vi "Launch Action - TDMS Writer Segmented.vi"(8 "error in (no error)":errorcluster, 9 "CAN Configurations":T2[](array[typedef]) {"Sample Rate (Hz)" format="%#_13g"}, 10 "DAQ AI Configurations":T1[](array[typedef]) {"Terminal Config" items=["Default"=-1, "RSE"=10083, "NRSE"=10078, "Differential"=10106, "Pseudodifferential"=12529]; "Min (V)" format="%#_13g"; "Max (V)" format="%#_13g"; "Sample Rate (Hz)" format="%#_13g"}, 11 "Log file path":path) -> (0 "error out":errorcluster)   [LabVIEW 2021, in "XNET-CAN-Signal-Logger.lvlib"]
uses:
  XNET-CAN-Signal-Logger.lvlib
  Typedef/Def-CAN Port Configuration.ctl
  Typedef/Def-DAQ AI Configuration.ctl
  Action - TDMS Writer.vi
  Global Variables.vi
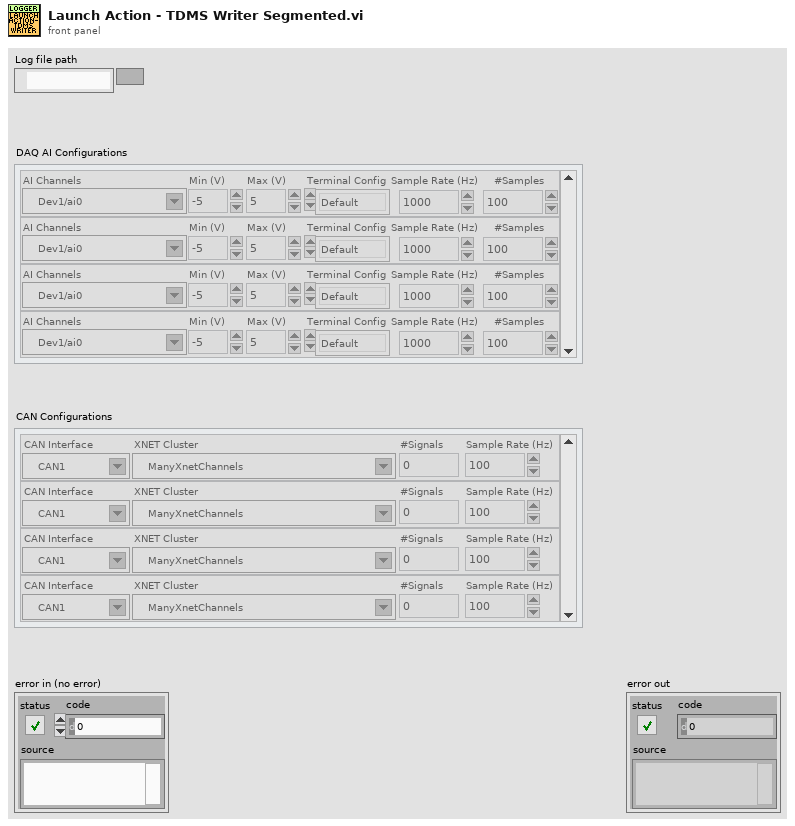
[diagram p1: front panel]
types:
  T1 = typedef "XNET-CAN-Signal-Logger.lvlib/Def-DAQ AI Configuration.ctl" = cluster{"AI Channels":tag, "Min (V)":dbl, "Max (V)":dbl, "Terminal Config":i32, "Sample Rate (Hz)":dbl, "#Samples":i32}
  T2 = typedef "XNET-CAN-Signal-Logger.lvlib/Def-CAN Port Configuration.ctl" = cluster{"CAN Interface":refnum<k21>, "XNET Cluster":refnum<k21>, "#Signals":i32, "Sample Rate (Hz)":dbl}
  T3 = enum16{"open", "open or create", "create or replace", "create", "open (read-only)"}
  T4 = typedef "XNET-CAN-Signal-Logger.lvlib/Def-FGV Data Type.ctl" = cluster{"DAQ AI Tasks":refnum<k21>[]}
  T5 = enum32{"Bad", "Idle", "Run top level", "Running"}
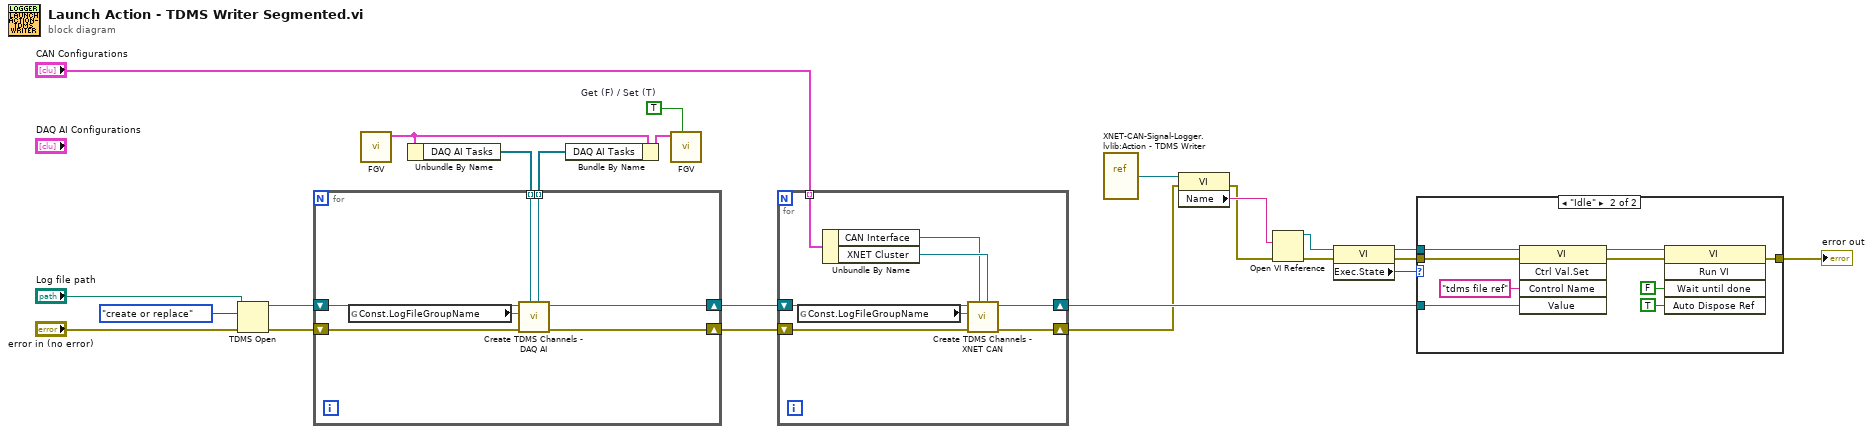
[diagram p0: block diagram]
diagram:
  w5 = TRUE  # Get (F) / Set (T)
  n1 = TDMS Open(8:"error in (no error)", 10:T3."create or replace" ("operation (0:open)"), 11:"Log file path") -> (0:w12:errorcluster, 3:w14:refnum<k34>)  [unwired: 4 in]
  n2 = call "FGV.vi"() -> ("data out"=w2:T4)  [unwired: 10 in, 1 out]
  n3 = Unbundle By Name(w2) -> ("DAQ AI Tasks"=w1:refnum<k21>[])
  n4 = for {
    shift-right: [w29] -> w13
    shift-left: w14 -> [w31]
    shift-right: [w28] -> w11
    shift-left: w12 -> [w26]
    tunnel: [w27] -> w3 mode=indexing
    tunnel: w1 -> [w25] mode=indexing
    n5 = global read "Global Variables.vi" "Const.LogFileGroupName"() -> (w30:string)
    n6 = call "Create TDMS Channels - DAQ AI.vi"("DAQ AI Task in"=w25, "error in (no error)"=w26, "group name in"=w30, "TDMS ref in"=w31) -> ("error out"=w28:errorcluster, "TDMS ref out"=w29:refnum<k34>, "DAQ AI Task out"=w27:refnum<k21>)  [unwired: 2 in, 3 out]
  }
  n7 = Bundle By Name(cluster=w2, "DAQ AI Tasks"=w3) -> (w4:T4)
  n8 = call "FGV.vi"("Get (F) / Set (T)"=w5, "data in"=w4) -> ()  [unwired: 8 in, 2 out]
  n9 = for {
    tunnel: "CAN Configurations" -> [w39] mode=indexing
    shift-right: [w34] -> w18
    shift-left: w13 -> [w36]
    shift-right: [w32] -> w16
    shift-left: w11 -> [w33]
    n10 = global read "Global Variables.vi" "Const.LogFileGroupName"() -> (w35:string)
    n11 = Unbundle By Name(w39) -> ("CAN Interface"=w37:refnum<k21>, "XNET Cluster"=w38:refnum<k21>)
    n12 = call "Create TDMS Channels - XNET CAN.vi"("XNET Cluster"=w38, "CAN Interface"=w37, "error in (no error)"=w33, "group name in"=w35, "TDMS ref in"=w36) -> ("error out"=w32:errorcluster, "TDMS ref out"=w34:refnum<k34>)  [unwired: 2 in, 3 out]
  }
  n13 = vi-ref "XNET-CAN-Signal-Logger.lvlib:Action - TDMS Writer.vi"() -> (w24:refnum<vi>)
  n14 = property class="VI"(reference=w24, error in=w16) -> (error out=w22:errorcluster, "Name"=w23:string)  [unwired: 1 out]
  n15 = Open VI Reference(vi path=w23, error in (no error)=w22) -> (vi reference=w21:refnum<vi>, error out=w9:errorcluster)  [unwired: 4 in]
  n16 = property class="VI"(reference=w21, error in=w9) -> (reference out=w8:refnum<vi>, error out=w7:errorcluster, "Exec.State"=w6:T5)
  n17 = case shown="\"Idle\"" w6 {
    tunnel: w18 -> [_ w46]
    tunnel: [w40 w41] -> w10
    tunnel: w8 -> [_ w43]
    tunnel: w7 -> [w40 w42]
    frame Default {
    }
    frame "Idle" {
      n18 = invoke class="VI" method="Ctrl Val.Set"(reference=w43, error in=w42, "Control Name"="tdms file ref", "Value"=w46) -> (reference out=w45:refnum<vi>, error out=w44:errorcluster)  [unwired: 1 in, 3 out]
      n19 = invoke class="VI" method="Run VI"(reference=w45, error in=w44, "Wait until done"=FALSE ("Wait Until Done"), "Auto Dispose Ref"=TRUE ("Auto Dispose Reference")) -> (error out=w41:errorcluster)  [unwired: 1 in, 4 out]
    }
  }
  "error out" <- w10
